vi "ActorPlugin-DatabaseManipulation.vi"(0 "FTW Actor Instance Configuration":string="{\n  \"Identity\": \"ActorName\",\n  \"InboxAddress\": \"tcp://127.0.0.1:*\",\n  \"PublisherAddress\": \"tcp://127.0.0.1:*\",\n  \"DebugEnableInboxLogging\": false,\n  \"DebugEnableJobLogging\": false,\n  \"DebugShowPanel\": false\n}") -> (15 "Error":errorcluster)   [LabVIEW 2013]
uses:
  ftw-dataflow/Actor/src/Instance/FTW-ActorInstance.lvclass
  ftw-dataflow/Actor/src/Message/Request/FTW-Message-IncomingRequest.lvclass
  PCert-Container/ERP-ConfigPageNewFeather/PCert-ConfigPageNF.lvclass
panel:
  # "Inputs"
  # "Outputs"
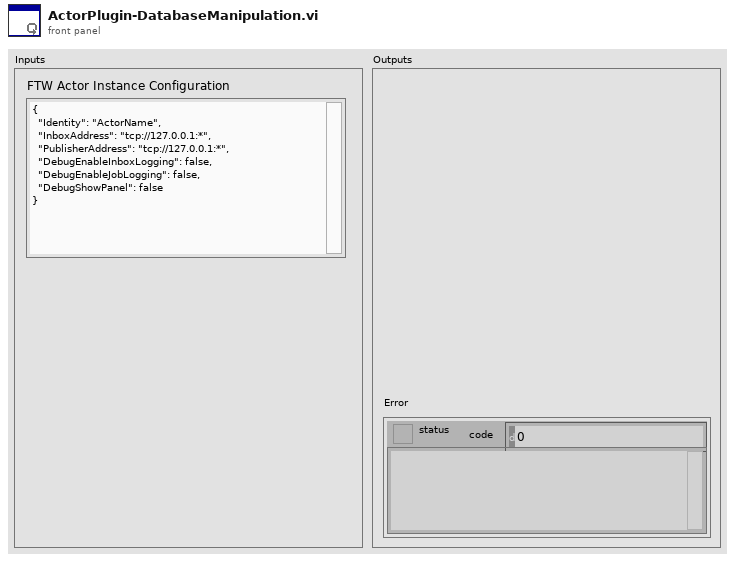
[diagram p1: front panel]
types:
  T1 = cluster{"Incoming Requests":refnum<event-registration>, "Additional Registration Types":refnum<event-registration>}
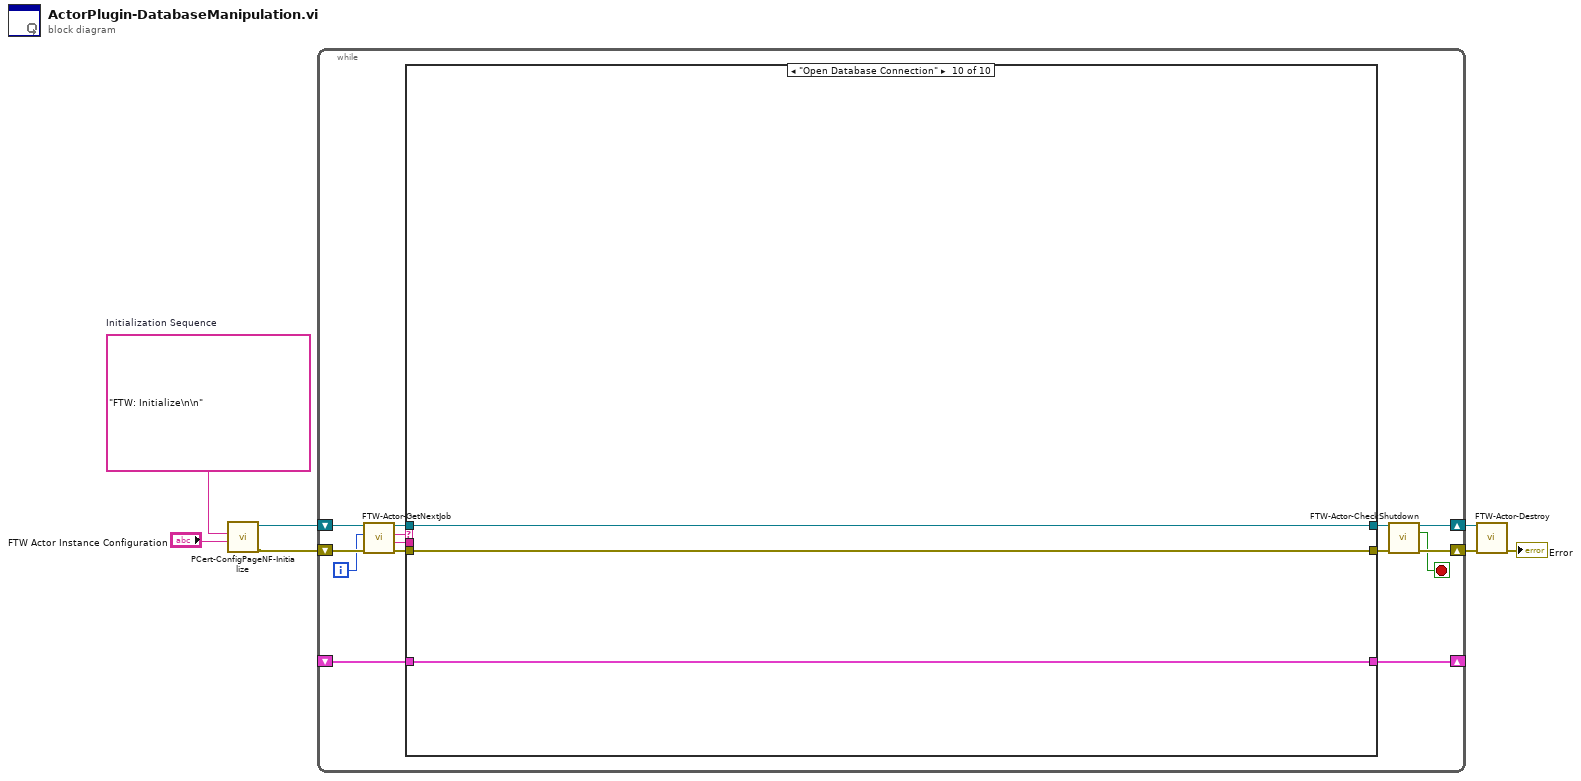
[diagram p0: block diagram]
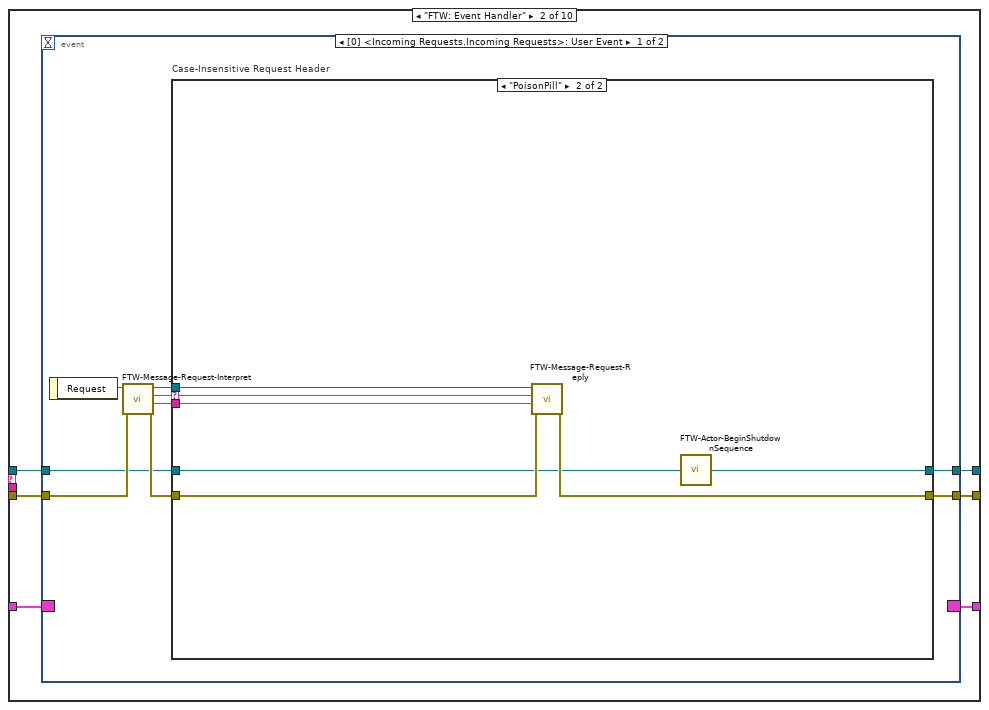
[diagram p3: hidden frame]
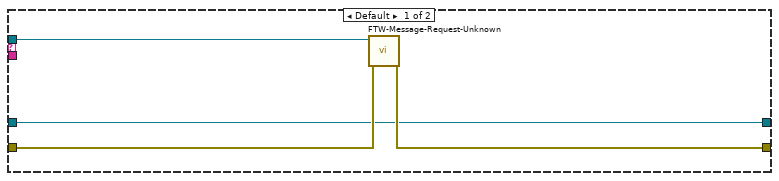
[diagram p4: hidden frame]
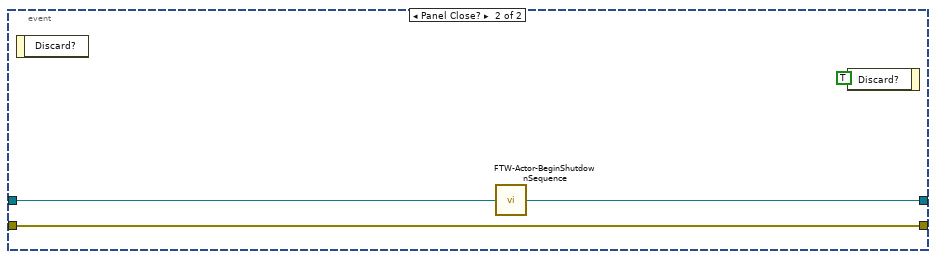
[diagram p5: hidden frame]
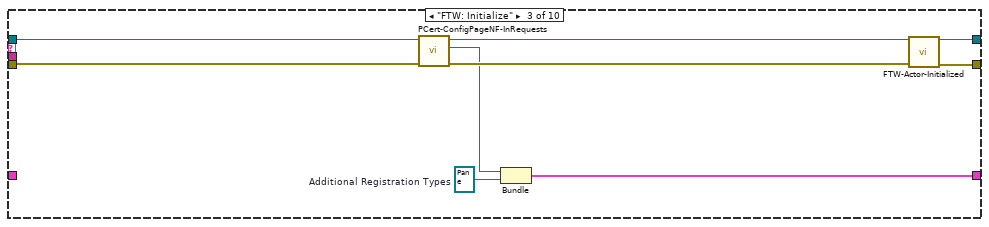
[diagram p6: hidden frame]
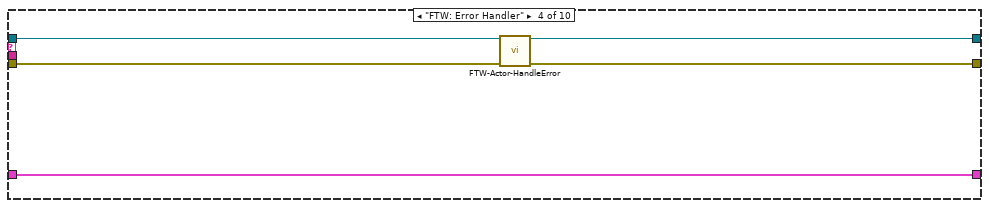
[diagram p7: hidden frame]
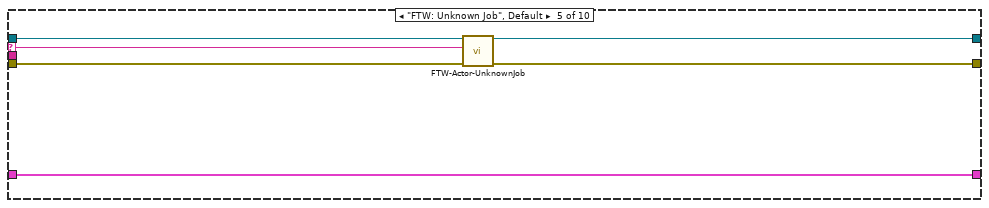
[diagram p8: hidden frame]
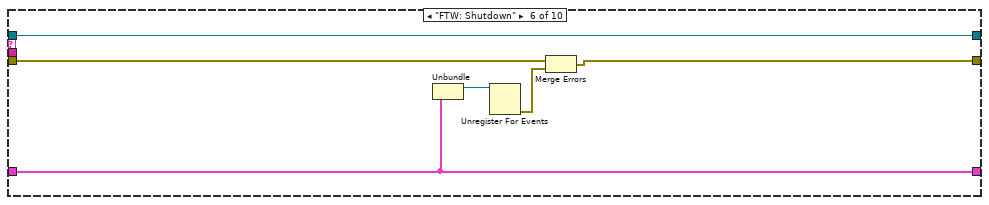
[diagram p9: hidden frame]
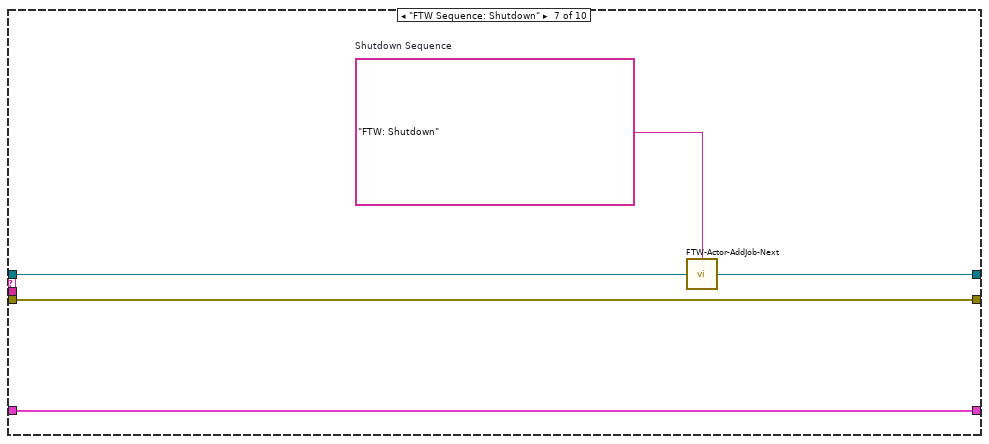
[diagram p10: hidden frame]
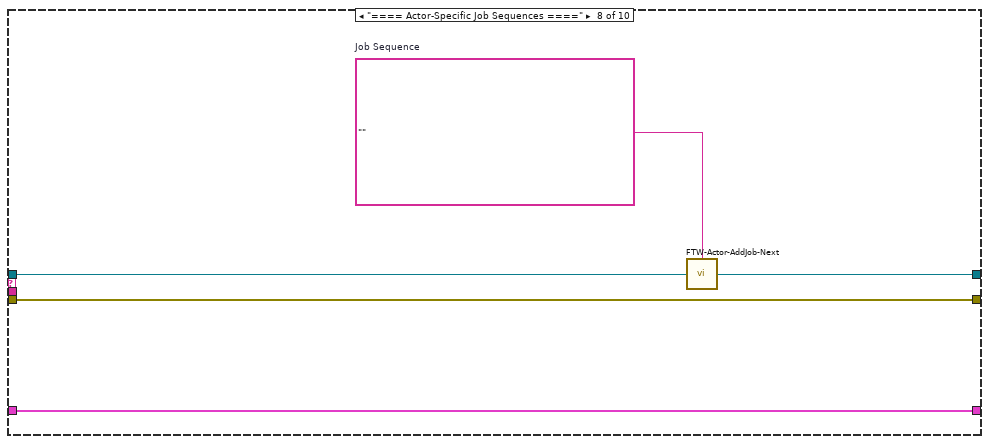
[diagram p11: hidden frame]
diagram:
  w4 = "FTW: Initialize\n\n"  # Initialization Sequence
  n1 = call-dynamic "PCert-ConfigPageNF-Initialize.vi"("FTW Actor Instance Configuration"="FTW Actor Instance Configuration", "Initialization Job Sequence"=w4) -> ("error out"=w2:errorcluster, "ERP-ConfigPageNF out"=w3:refnum<class "PCert-ConfigPageNF.lvclass">)  [unwired: 8 in]
  n2 = while {
    shift-right: [w11] -> w6
    shift-left: w2 -> [w18]
    shift-right: [w8] -> _
    shift-left: _ -> [w21]
    shift-right: [w13] -> w7
    shift-left: w3 -> [w20]
    i -> [w9]
    stop <- w10 stop-if-true
    n3 = call "FTW-Actor-GetNextJob.vi"("error in"=w18, "Jobs Performed"=w9, "FTW Actor Instance"=w20) -> ("error out"=w17:errorcluster, "Job Data"=w15:string, "Job Name"=w16:string, "FTW Actor Instance out"=w19:refnum<class "PCert-ConfigPageNF.lvclass">)  [unwired: 5 in]
    n4 = case shown="\"Open Database Connection\"" w16 {
      selector: w16 -> [_ _ _ _ w69 _ _ _ _ _]
      tunnel: [w23 w30 w62 w64 w72 w78 w84 w89 w93 w96] -> w12
      tunnel: w17 -> [w23 w29 w59 w66 w73 w75 w84 w89 w93 w96]
      tunnel: w21 -> [w24 w25 _ w68 w74 w80 w85 w90 w92 w95]
      tunnel: [w24 w28 w55 w68 w74 w80 w85 w90 w92 w95] -> w8
      tunnel: w15 -> [_ _ _ _ _ _ _ _ _ _]
      tunnel: [w22 w27 w63 w65 w70 w76 w82 w87 w91 w94] -> w14
      tunnel: w19 -> [w22 w26 w61 w67 w71 w76 w83 w88 w91 w94]
      frame "==== Featherweight Framework Jobs ====" {
      }
      frame "FTW: Event Handler" {
        n5 = event shown="[0] <Incoming Requests.Incoming Requests>: User Event" {
          selector: w25 -> [_ _]
          dyn-events: [_ _] -> w28
          timeout: _ -> [_ _]
          tunnel: [w36 w53] -> w30
          tunnel: w29 -> [w37 w53]
          tunnel: [w35 w51] -> w27
          tunnel: w26 -> [w34 w52]
          event User Event {
            n6 = event-data() -> ("Request"=w38:refnum<class "FTW-Message-IncomingRequest.lvclass">)  [unwired: 1 in]
            n7 = call "FTW-Message-Request-Interpret.vi"("error in"=w37, "FTW Incoming Request"=w38) -> ("error out"=w39:errorcluster, "Request Body"=w32:string, "Request Header"=w33:string, "FTW Incoming Request out"=w31:refnum<class "FTW-Message-IncomingRequest.lvclass">)  [unwired: 6 in]
            n8 = case "Case-Insensitive Request Header" shown="\"PoisonPill\"" w33 {
              selector: w33 -> [_ w45]
              tunnel: [w42 w47] -> w36
              tunnel: w39 -> [w43 w48]
              tunnel: [w40 w50] -> w35
              tunnel: w34 -> [w40 w46]
              tunnel: w32 -> [_ w44]
              tunnel: w31 -> [w41 w49]
              frame Default {
                n9 = call "FTW-Message-Request-Unknown.vi"("error in"=w43, "FTW Incoming Request"=w41) -> ("error out"=w42:errorcluster)  [unwired: 9 in]
              }
              frame "PoisonPill" {
                n10 = call "FTW-Message-Request-Reply.vi"("error in"=w48, "Response Body"=w44, "Response Header"=w45, "FTW Incoming Request"=w49) -> ("error out"=w47:errorcluster)  [unwired: 6 in, 1 out]
                n11 = call "FTW-Actor-BeginShutdownSequence.vi"("FTW Actor Instance"=w46) -> ("FTW Actor Instance out"=w50:refnum<class "PCert-ConfigPageNF.lvclass">)  [unwired: 3 in]
              }
            }
          }
          event Panel Close? {
            n12 = event-data() -> ()  [unwired: 1 in, 1 out]
            n13 = call "FTW-Actor-BeginShutdownSequence.vi"("FTW Actor Instance"=w52) -> ("FTW Actor Instance out"=w51:refnum<class "PCert-ConfigPageNF.lvclass">)  [unwired: 3 in]
            n14 = event-data("Discard?"=TRUE) -> ()  [unwired: 1 in, 1 out]
          }
        }
      }
      frame "FTW: Initialize" {
        w57 = refnum<event-registration> refnum  # Additional Registration Types
        n15 = call "PCert-ConfigPageNF-InRequests.vi"("error in (no error)"=w59, "ERP-ConfigPageNF in"=w61) -> ("error out"=w58:errorcluster, "Incoming Requests"=w56:refnum<event-registration>, "ERP-ConfigPageNF out"=w60:refnum<class "PCert-ConfigPageNF.lvclass">)  [unwired: 7 in]
        n16 = Bundle("Incoming Requests"=w56, "Additional Registration Types"=w57) -> (w55:T1)  [unwired: 1 in]
        n17 = call-dynamic "FTW-Actor-Initialized.vi"("FTW Actor Instance"=w60, "error in"=w58) -> ("FTW Actor Instance out"=w63:refnum<class "PCert-ConfigPageNF.lvclass">, "error out"=w62:errorcluster)  [unwired: 12 in]
      }
      frame "FTW: Error Handler" {
        n18 = call-dynamic "FTW-Actor-HandleError.vi"("FTW Actor Instance"=w67, "error in"=w66) -> ("FTW Actor Instance out"=w65:refnum<class "PCert-ConfigPageNF.lvclass">, "error out"=w64:errorcluster)  [unwired: 11 in, 1 out]
      }
      frame "FTW: Unknown Job", Default {
        n19 = call-dynamic "FTW-Actor-UnknownJob.vi"("FTW Actor Instance"=w71, "Unknown Job"=w69, "error in"=w73) -> ("FTW Actor Instance out"=w70:refnum<class "PCert-ConfigPageNF.lvclass">, "error out"=w72:errorcluster)  [unwired: 11 in]
      }
      frame "FTW: Shutdown" {
        n20 = Unbundle(w80) -> ("Incoming Requests"=w79:refnum<event-registration>)  [unwired: 1 out]
        n21 = Unregister For Events(event registration refnum=w79) -> (error out=w77:errorcluster)  [unwired: 1 in]
        n22 = Merge Errors(w75, w77) -> (w78:errorcluster)
      }
      frame "FTW Sequence: Shutdown" {
        w81 = "FTW: Shutdown"  # Shutdown Sequence
        n23 = call "FTW-Actor-AddJob-Next.vi"("Add Next in Job Queue"=w81, "FTW Actor Instance"=w83) -> ("FTW Actor Instance out"=w82:refnum<class "PCert-ConfigPageNF.lvclass">)  [unwired: 2 in]
      }
      frame "==== Actor-Specific Job Sequences ====" {
        w86 = ""  # Job Sequence
        n24 = call "FTW-Actor-AddJob-Next.vi"("Add Next in Job Queue"=w86, "FTW Actor Instance"=w88) -> ("FTW Actor Instance out"=w87:refnum<class "PCert-ConfigPageNF.lvclass">)  [unwired: 2 in]
      }
      frame "==== Actor-Specific Jobs ====" {
      }
      frame "Open Database Connection" {
      }
    }
    n25 = call "FTW-Actor-CheckShutdown.vi"("FTW Actor Instance"=w14, "error in"=w12) -> ("FTW Actor Instance out"=w13:refnum<class "PCert-ConfigPageNF.lvclass">, "Shutdown?"=w10:bool, "error out"=w11:errorcluster)  [unwired: 11 in]
  }
  n26 = call-dynamic "FTW-Actor-Destroy.vi"("FTW Actor Instance"=w7, "error in"=w6) -> ("error out"=→"Error":errorcluster)  [unwired: 13 in]
